vi "Shift Register.vi"() -> ()   [LabVIEW 2015]
panel:
  out "Numeric 2":dbl
  in  "stop":bool
  in  "s":bool
  in  "Numeric":dbl
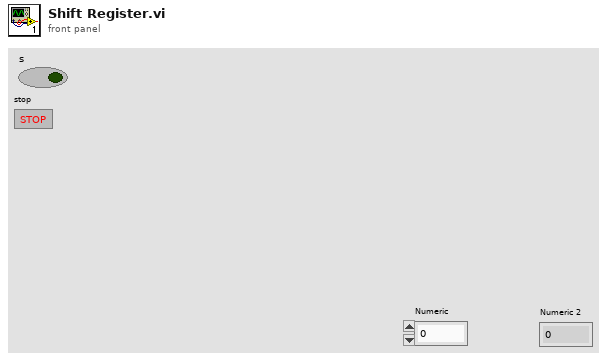
[diagram p1: front panel]
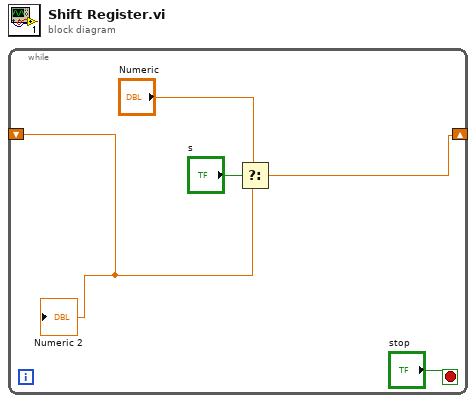
[diagram p0: block diagram]
diagram:
  n1 = while {
    shift-right: [w5] -> _
    shift-left: _ -> [w1]
    stop <- "stop" stop-if-true
    n2 = Select(t="Numeric", s="s", f=w1) -> (s? t:f=w5:dbl)
    "Numeric 2" <- w1
  }
